vi "ep_Read Analog Channel Info.vi"(8 "error in (no error)":errorcluster, 11 "task in":T2={"file refnums"=[], "Data Object"=refnum, "config info"={"station_name"="", "rec_dev_id"="", "rev_year"=1999.0, "TT"=0, "##A"=0, "##D"=0, "analog channel info"=[], "status channel info"=[], "lf"=50.0, "nrates"=0, "samp info"=[], "initial timestamp"=timestamp(0 s since 1904-01-01), "trigger timestamp"=timestamp(0 s since 1904-01-01), "ft"=enum."Binary", "timemult"=1.0}, "public inf content"={"Source"="", "Record Type"=enum."Unknown", "Phase ID"="", "Event Description"="", "Device ID"="", "Distance of Fault"=-1.0, "Distance Unit"=enum."Miles", "Max_Current"=inf, "Min_Current"=-inf, "Max_Voltage"=inf, "Min_Voltage"=-inf, "EventNoteCount"=0, "Event Information"=[]}, "private inf content"=[], "internal buffers"={"start index"=1, "config to public inf"=enum."disabled", "static config info"="", "static file_des record inf"="", "static file_des channel inf"="", "public inf"="", "private inf"=""}} {"public inf content"."Event Information"."min sample number" max=9999999999; "public inf content"."Event Information"."max sample number" max=9999999999; "config info"."nrates" max=999; "config info"."status channel info"."Dn" min=1 max=999999; "config info"."analog channel info"."An" min=1 max=999999; "config info"."trigger timestamp" format="%<%H:%M:%S%6u\n%d/%m/%Y>T"; "config info"."initial timestamp" format="%<%H:%M:%S%6u\n%d/%m/%Y>T"; "config info"."##D" max=999999; "config info"."##A" max=999999; "config info"."TT" min=1 max=999999; "config info"."rev_year" min=1999.0 max=1999.0}) -> (0 "error out":errorcluster, 2 "analog channel info":T1[](array[typedef]), 3 "task out":T2={"file refnums"=[], "Data Object"=refnum, "config info"={"station_name"="", "rec_dev_id"="", "rev_year"=1999.0, "TT"=0, "##A"=0, "##D"=0, "analog channel info"=[], "status channel info"=[], "lf"=50.0, "nrates"=0, "samp info"=[], "initial timestamp"=timestamp(0 s since 1904-01-01), "trigger timestamp"=timestamp(0 s since 1904-01-01), "ft"=enum."Binary", "timemult"=1.0}, "public inf content"={"Source"="", "Record Type"=enum."Unknown", "Phase ID"="", "Event Description"="", "Device ID"="", "Distance of Fault"=-1.0, "Distance Unit"=enum."Miles", "Max_Current"=inf, "Min_Current"=-inf, "Max_Voltage"=inf, "Min_Voltage"=-inf, "EventNoteCount"=0, "Event Information"=[]}, "private inf content"=[], "internal buffers"={"start index"=1, "config to public inf"=enum."disabled", "static config info"="", "static file_des record inf"="", "static file_des channel inf"="", "public inf"="", "private inf"=""}} {"public inf content"."Event Information"."min sample number" max=9999999999; "public inf content"."Event Information"."max sample number" max=9999999999; "config info"."nrates" max=999; "config info"."status channel info"."Dn" min=1 max=999999; "config info"."analog channel info"."An" min=1 max=999999; "config info"."trigger timestamp" format="%<%H:%M:%S%6u\n%d/%m/%Y>T"; "config info"."initial timestamp" format="%<%H:%M:%S%6u\n%d/%m/%Y>T"; "config info"."##D" max=999999; "config info"."##A" max=999999; "config info"."TT" min=1 max=999999; "config info"."rev_year" min=1999.0 max=1999.0})   [LabVIEW 2014, in "NI_EP_COMTRADE.lvlib"]
uses:
  <vilib>/addons/Electrical Power/File IO/NI_EP_COMTRADE.lvlib
  <vilib>/addons/Electrical Power/File IO/COMTRADE/typedefs/ep_Task.ctl
  <vilib>/addons/Electrical Power/File IO/COMTRADE/typedefs/ep_Config Info.ctl
  <vilib>/addons/Electrical Power/File IO/COMTRADE/typedefs/ep_Analog Channel Info.ctl
  <vilib>/addons/Electrical Power/File IO/COMTRADE/typedefs/ep_Status Channel Info.ctl
  <vilib>/addons/Electrical Power/File IO/COMTRADE/typedefs/ep_File Format.ctl
  <vilib>/addons/Electrical Power/File IO/COMTRADE/typedefs/ep_Public Inf Content.ctl
  <vilib>/addons/Electrical Power/File IO/COMTRADE/typedefs/ep_Public Event Inf.ctl
  <vilib>/addons/Electrical Power/File IO/COMTRADE/typedefs/ep_Private Inf Content.ctl
  <vilib>/addons/Electrical Power/File IO/COMTRADE/typedefs/ep_Analog Channel Info (UI).ctl
  <vilib>/Platform/storage/Storage.llb/Get Property (Storage Refnums).vi
  <vilib>/Platform/storage/Storage.llb/Get Property (I32).vi
  <vilib>/Platform/storage/Storage.llb/Get Property (String).vi
  <vilib>/Platform/storage/Storage.llb/Get Property (SGL).vi
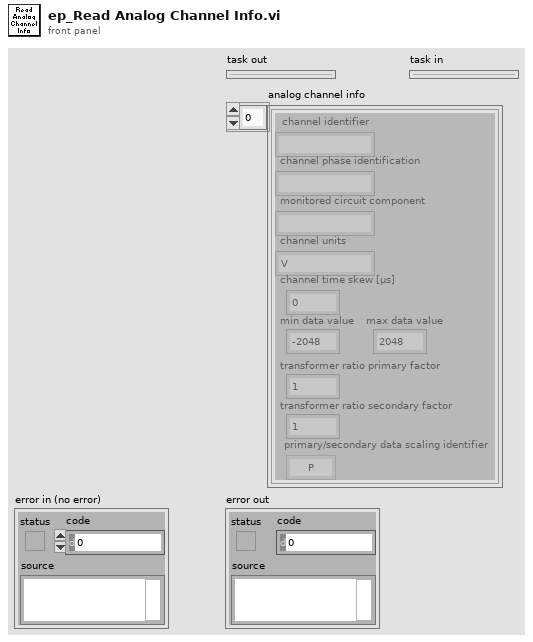
[diagram p1: front panel]
types:
  T1 = typedef "NI_EP_COMTRADE.lvlib/ep_Analog Channel Info (UI).ctl" = cluster{"channel identifier":string, "channel phase identification":string, "monitored circuit component":string, "channel units":string, "channel time skew [µs]":sgl, "min data value":sgl, "max data value":sgl, "transformer ratio primary factor":sgl, "transformer ratio secondary factor":sgl, "primary/secondary data scaling identifier":enum16{"P", "S"}}
  T2 = typedef "NI_EP_COMTRADE.lvlib/ep_Task.ctl" = cluster{"file refnums":refnum<file>[], "Data Object":refnum<k20>, "config info":T3, "public inf content":T7, "private inf content":T9, "internal buffers":cluster{"start index":u32, "config to public inf":enum16{"disabled", "enabled", "buffered"}, "static config info":string, "static file_des record inf":string, "static file_des channel inf":string, "public inf":string, "private inf":string}}
  T3 = typedef "NI_EP_COMTRADE.lvlib/ep_Config Info.ctl" = cluster{"station_name":string, "rec_dev_id":string, "rev_year":dbl, "TT":u32, "##A":u32, "##D":u32, "analog channel info":T4[], "status channel info":T5[], "lf":sgl, "nrates":u16, "samp info":cluster{"samp":sgl, "endsamp":u32}[], "initial timestamp":timestamp, "trigger timestamp":timestamp, "ft":T6, "timemult":sgl}
  T4 = typedef "NI_EP_COMTRADE.lvlib/ep_Analog Channel Info.ctl" = cluster{"An":u32, "ch_id":string, "ph":string, "ccbm":string, "uu":string, "a":sgl, "b":sgl, "skew":sgl, "min":i32, "max":i32, "primary":sgl, "secondary":sgl, "PS":enum16{"P", "S"}}
  T5 = typedef "NI_EP_COMTRADE.lvlib/ep_Status Channel Info.ctl" = cluster{"Dn":u32, "ch_id":string, "ph":string, "ccbm":string, "Y":bool}
  T6 = typedef "NI_EP_COMTRADE.lvlib/ep_File Format.ctl" = enum16{"ASCII", "Binary"}
  T7 = typedef "NI_EP_COMTRADE.lvlib/ep_Public Inf Content.ctl" = cluster{"Source":string, "Record Type":enum16{"Fault", "Unknown", "Misoperation", "Close", "Trip", "Reclose", "Power swing", "Simulation"}, "Phase ID":string, "Event Description":string, "Device ID":string, "Distance of Fault":dbl, "Distance Unit":enum16{"Miles", "Kilometers", "Percent of line", "Percent of setting", "Ohms"}, "Max_Current":dbl, "Min_Current":dbl, "Max_Voltage":dbl, "Min_Voltage":dbl, "EventNoteCount":u32, "Event Information":T8[]}
  T8 = typedef "NI_EP_COMTRADE.lvlib/ep_Public Event Inf.ctl" = cluster{"channel number":u32, "max value":dbl, "min value":dbl, "max sample number":u64, "min sample number":u64, "max sample text":string[], "min sample text":string[]}
  T9 = typedef "NI_EP_COMTRADE.lvlib/ep_Private Inf Content.ctl" = cluster{"Section Header":string, "Entry Names":string[], "Entry Values":string[]}[]
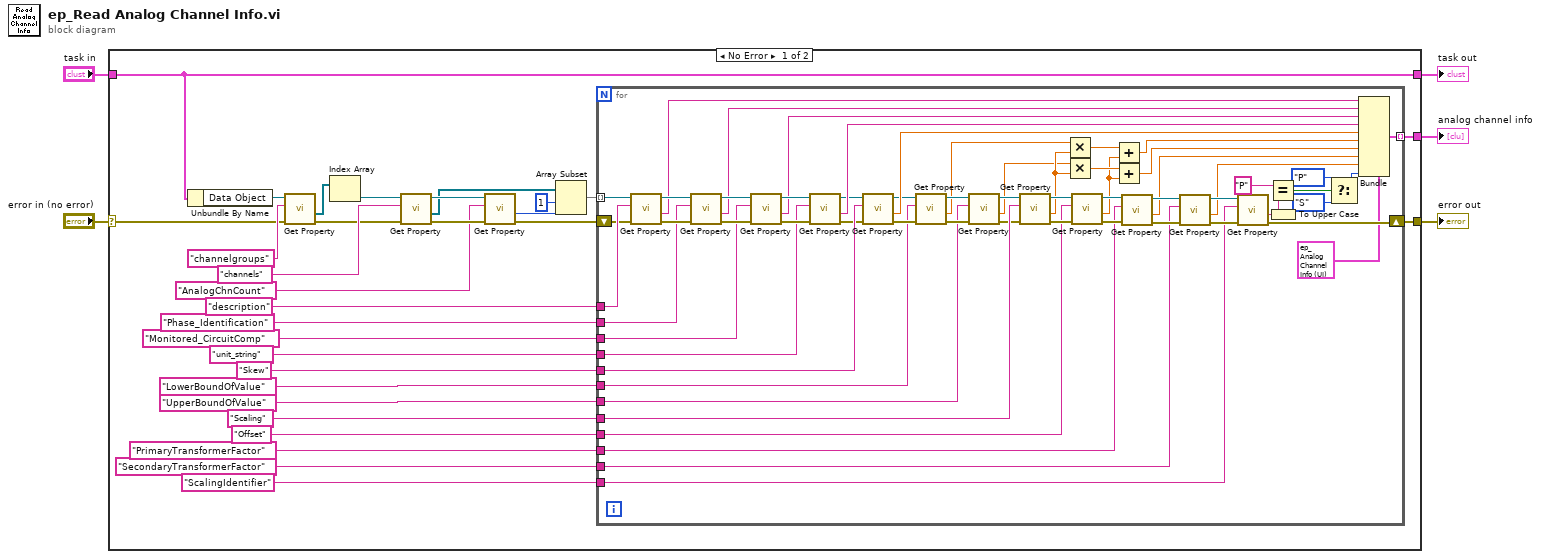
[diagram p0: block diagram]
diagram:
  n1 = case shown="No Error" "error in (no error)" {
    selector: "error in (no error)" -> [w31 w98]
    tunnel: [w35 w97] -> w4
    tunnel: "task in" -> [w35 w97]
    tunnel: [w15 _] -> w2
    tunnel: [w7 w98] -> w1
    frame No Error {
      n2 = Unbundle By Name(w35) -> ("Data Object"=w34:refnum<k20>)
      n3 = call-poly <vilib>:"Get Property.vi"("error in (no error)"=w31, "Property name"="channelgroups", "storage refnum"=w34) -> ("error out"=w6:errorcluster, "Value"=w32:refnum<k20>[])  [unwired: 6 in, 1 out]
      n4 = Index Array(array=w32) -> (element=w30:refnum<k20>)  [unwired: 1 in]
      n5 = call-poly <vilib>:"Get Property.vi"("error in (no error)"=w6, "Property name"="channels", "storage refnum"=w30) -> ("error out"=w27:errorcluster, "Value"=w12:refnum<k20>[], "storage refnum out"=w28:refnum<k20>)  [unwired: 6 in]
      n6 = call-poly <vilib>:"Get Property.vi"("error in (no error)"=w27, "Property name"="AnalogChnCount", "storage refnum"=w28) -> ("error out"=w24:errorcluster, "Value"=w14:i32)  [unwired: 6 in, 1 out]
      n7 = Array Subset(array=w12, index=1, length=w14) -> (w13:refnum<k20>[])
      n8 = for {
        tunnel: w13 -> [w96] mode=indexing
        tunnel: "description" ("Property name") -> [w95]
        shift-right: [w73] -> w7
        shift-left: w24 -> [w94]
        tunnel: "Phase_Identification" ("Property name") -> [w91]
        tunnel: "Monitored_CircuitComp" ("Property name") -> [w88]
        tunnel: "unit_string" ("Property name") -> [w85]
        tunnel: "Skew" ("Property name") -> [w84]
        tunnel: "Scaling" ("Property name") -> [w83]
        tunnel: "Offset" ("Property name") -> [w76]
        tunnel: "PrimaryTransformerFactor" ("Property name") -> [w75]
        tunnel: "SecondaryTransformerFactor" ("Property name") -> [w74]
        tunnel: "ScalingIdentifier" ("Property name") -> [w70]
        tunnel: [w56] -> w15 mode=indexing
        tunnel: "LowerBoundOfValue" ("Property name") -> [w49]
        tunnel: "UpperBoundOfValue" ("Property name") -> [w48]
        n9 = call-poly <vilib>:"Get Property.vi"("error in (no error)"=w94, "Property name"=w95, "storage refnum"=w96) -> ("error out"=w93:errorcluster, "Value"=w64:string, "storage refnum out"=w92:refnum<k20>)  [unwired: 6 in]
        n10 = call-poly <vilib>:"Get Property.vi"("error in (no error)"=w93, "Property name"=w91, "storage refnum"=w92) -> ("error out"=w90:errorcluster, "Value"=w63:string, "storage refnum out"=w89:refnum<k20>)  [unwired: 6 in]
        n11 = call-poly <vilib>:"Get Property.vi"("error in (no error)"=w90, "Property name"=w88, "storage refnum"=w89) -> ("error out"=w86:errorcluster, "Value"=w62:string, "storage refnum out"=w87:refnum<k20>)  [unwired: 6 in]
        n12 = call-poly <vilib>:"Get Property.vi"("error in (no error)"=w86, "Property name"=w85, "storage refnum"=w87) -> ("error out"=w38:errorcluster, "Value"=w61:string, "storage refnum out"=w39:refnum<k20>)  [unwired: 6 in]
        n13 = call-poly <vilib>:"Get Property.vi"("error in (no error)"=w38, "Property name"=w84, "storage refnum"=w39) -> ("error out"=w54:errorcluster, "Value"=w60:sgl, "storage refnum out"=w55:refnum<k20>)  [unwired: 6 in]
        n14 = call-poly <vilib>:"Get Property.vi"("error in (no error)"=w54, "Property name"=w49, "storage refnum"=w55) -> ("error out"=w52:errorcluster, "Value"=w47:sgl, "storage refnum out"=w53:refnum<k20>)  [unwired: 6 in]
        n15 = call-poly <vilib>:"Get Property.vi"("error in (no error)"=w52, "Property name"=w48, "storage refnum"=w53) -> ("error out"=w50:errorcluster, "Value"=w44:sgl, "storage refnum out"=w51:refnum<k20>)  [unwired: 6 in]
        n16 = call-poly <vilib>:"Get Property.vi"("error in (no error)"=w50, "Property name"=w83, "storage refnum"=w51) -> ("error out"=w77:errorcluster, "Value"=w45:sgl, "storage refnum out"=w78:refnum<k20>)  [unwired: 6 in]
        n17 = Multiply(x=w47, y=w45) -> (x*y=w46:sgl)
        n18 = Multiply(x=w44, y=w45) -> (x*y=w43:sgl)
        n19 = call-poly <vilib>:"Get Property.vi"("error in (no error)"=w77, "Property name"=w76, "storage refnum"=w78) -> ("error out"=w82:errorcluster, "Value"=w41:sgl, "storage refnum out"=w81:refnum<k20>)  [unwired: 6 in]
        n20 = Add(x=w46, y=w41) -> (x+y=w42:sgl)
        n21 = Add(x=w43, y=w41) -> (x+y=w40:sgl)
        n22 = call-poly <vilib>:"Get Property.vi"("error in (no error)"=w82, "Property name"=w75, "storage refnum"=w81) -> ("error out"=w80:errorcluster, "Value"=w59:sgl, "storage refnum out"=w79:refnum<k20>)  [unwired: 6 in]
        n23 = call-poly <vilib>:"Get Property.vi"("error in (no error)"=w80, "Property name"=w74, "storage refnum"=w79) -> ("error out"=w71:errorcluster, "Value"=w58:sgl, "storage refnum out"=w72:refnum<k20>)  [unwired: 6 in]
        n24 = call-poly <vilib>:"Get Property.vi"("error in (no error)"=w71, "Property name"=w70, "storage refnum"=w72) -> ("error out"=w73:errorcluster, "Value"=w69:string)  [unwired: 6 in, 1 out]
        n25 = To Upper Case(1:w69) -> (0:w37:string)
        n26 = Equal?(x="P", y=w37) -> (x = y?=w67:bool)
        n27 = Select(t=enum16{"P", "S"}."P" ("PS"), s=w67, f=enum16{"P", "S"}."S" ("PS")) -> (s? t:f=w57:enum16{"P", "S"})
        n28 = Bundle(cluster=T1 {"channel identifier"="", "channel phase identification"="", "monitored circuit component"="", "channel units"="", "channel time skew [µs]"=0.0, "min data value"=0.0, "max data value"=0.0, "transformer ratio primary factor"=0.0, "transformer ratio secondary factor"=0.0, "primary/secondary data scaling identifier"=enum."P"}, "channel identifier"=w64, "channel phase identification"=w63, "monitored circuit component"=w62, "channel units"=w61, "channel time skew [µs]"=w60, "min data value"=w42, "max data value"=w40, "transformer ratio primary factor"=w59, "transformer ratio secondary factor"=w58, "primary/secondary data scaling identifier"=w57) -> (w56:T1)
      }
    }
    frame Error {
    }
  }
  "error out" <- w1
  "task out" <- w4
  "analog channel info" <- w2
